vi "GT Load Ext Config.vi"(8 "error in (no error)":errorcluster caption="错误输入（无错误）", 10 "pFileName":string, 11 "cardNum":i16) -> (0 "error out":errorcluster caption="错误输出", 2 "pFileName out":string, 3 "function return":i16)   [LabVIEW 2014, in "gts.lvlib"]
doc: "GT_API GT_LoadExtConfig(short cardNum,char *pFileName);"
uses:
  gts.lvlib
  gts.dll
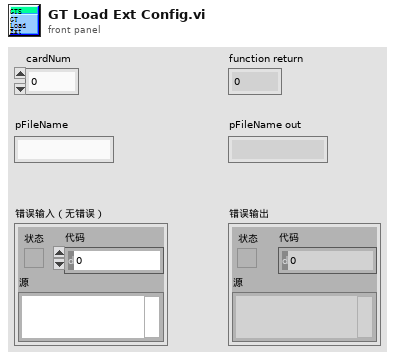
[diagram p1: front panel]
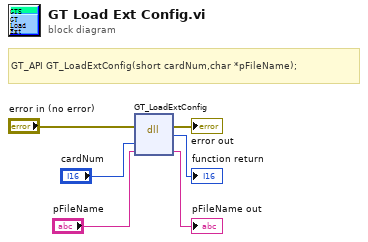
[diagram p0: block diagram]
diagram:
  # "GT_API GT_LoadExtConfig(short cardNum,char *pFileName);"
  n1 = dll-call lib="PTH2kabs D固高科技资料LABVIEWlabview 例程.多卡库-控制卡基本运动例程(labview)gts.*" fn="GT_LoadExtConfig"(error in="error in (no error)", "cardNum"="cardNum", "pFileName"="pFileName") -> (error out=→"error out":errorcluster, →"function return":i16, "pFileName"=→"pFileName out":string)  [unwired: 3 in, 1 out]
